vi "main_display.vi"() -> ()   [LabVIEW 2021]
uses:
  <vilib>/Instr/_visa.llb/VISA Configure Serial Port (Instr).vi
  <vilib>/Utility/file.llb/Write Delimited Spreadsheet (DBL).vi
panel:
  out "read buffer":string
  in  "Save Data":bool
  out "Sensor 8":dbl(slide) scale=0.0..10.0
  out "Sensor 7":dbl(slide) scale=0.0..10.0
  out "Sensor 6":dbl(slide) scale=0.0..10.0
  out "Sensor 5":dbl(slide) scale=0.0..10.0
  out "Sensor 4":dbl(slide) scale=0.0..10.0
  out "Sensor 3":dbl(slide) scale=0.0..10.0
  out "Sensor 2":dbl(slide) scale=0.0..10.0
  out "Sensor 1":dbl(slide) scale=0.0..10.0
  out "Output":dbl[](array[numeric])
  in  "file path (dialog if empty)":path
  out "Read time (ms)":u32
  in  "stop":bool
  in  "VISA resource name":refnum<visa-resource-name>
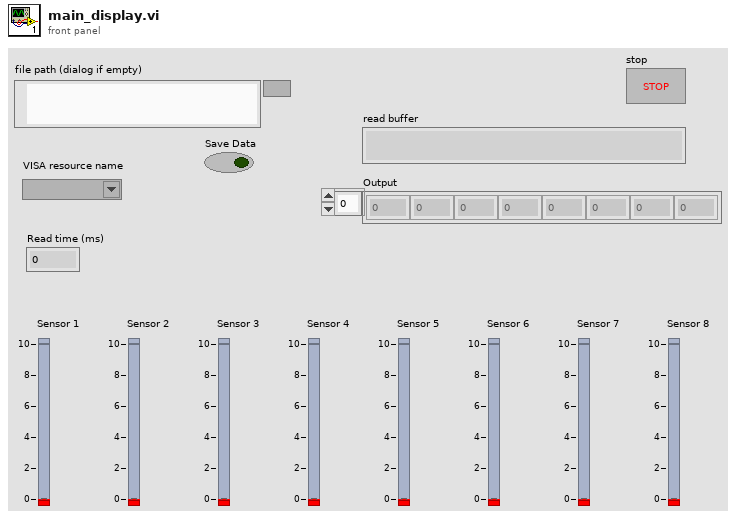
[diagram p1: front panel]
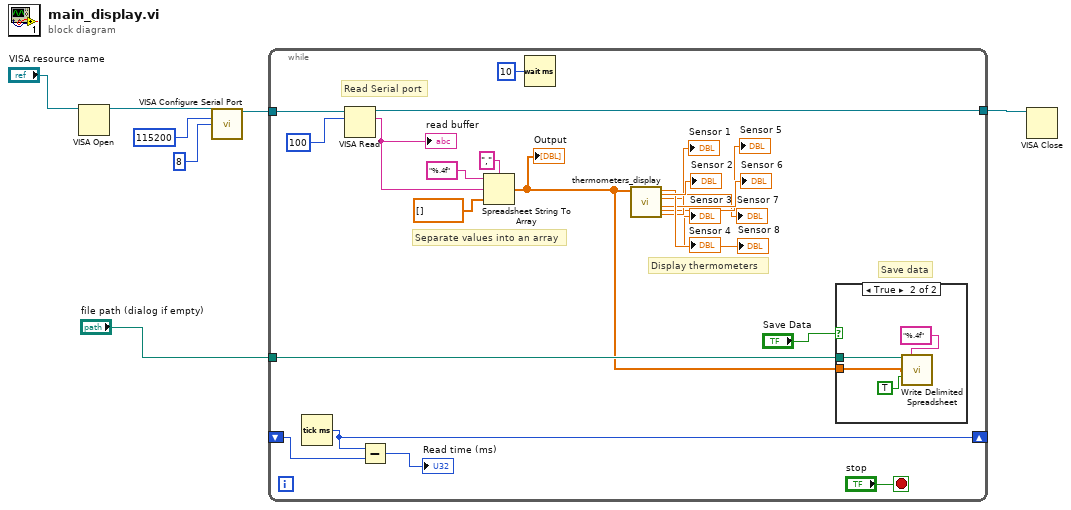
[diagram p0: block diagram]
diagram:
  n1 = VISA Open(VISA resource name="VISA resource name") -> (VISA resource name=w3:refnum<visa-resource-name>)  [unwired: 4 in, 1 out]
  n2 = call-poly "VISA Configure Serial Port"("VISA resource name"=w3, "baud rate (9600)"=u32 115200, "data bits (8)"=u16 8) -> ("VISA resource name out"=w5:refnum<visa-resource-name>)  [unwired: 11 in, 1 out]
  n3 = while {
    tunnel: w5 -> [w27]
    tunnel: [w28] -> w4
    shift-right: [w25] -> _
    shift-left: _ -> [w24]
    tunnel: "file path (dialog if empty)" -> [w22]
    stop <- "stop" stop-if-true
    # "Display thermometers"
    # "Save data"
    # "Separate values into an array"
    # "Read Serial port"
    n4 = Tick Count (ms)() -> (millisecond timer value=w25:u32)
    n5 = VISA Read(VISA resource name=w27, byte count=u32 100) -> (VISA resource name out=w28:refnum<visa-resource-name>, read buffer=w21:string)  [unwired: 1 in, 2 out]
    "read buffer" <- w21
    n6 = Subtract(x=w25, y=w24) -> (x-y=→"Read time (ms)":u32)
    n7 = Spreadsheet String To Array(delimiter (Tab)=",", format string="%.4f", spreadsheet string=w21, array type (2D Dbl)=dbl[] []) -> (array=w9:dbl[])
    "Output" <- w9
    n8 = Wait (ms)(milliseconds to wait=u32 10) -> ()  [unwired: 1 out]
    n9 = call "thermometers_display.vi"("array type (2D Dbl)"=w9) -> ("Sensor 1"=→"Sensor 1":dbl, "Sensor 6"=→"Sensor 6":dbl, "Sensor 4"=→"Sensor 4":dbl, "Sensor 8"=→"Sensor 8":dbl, "Sensor 5"=→"Sensor 5":dbl, "Sensor 2"=→"Sensor 2":dbl, "Sensor 3"=→"Sensor 3":dbl, "Sensor 7"=→"Sensor 7":dbl)  [unwired: 3 in]
    n10 = case shown="True" "Save Data" {
      tunnel: w22 -> [_ w32]
      tunnel: w9 -> [_ w31]
      frame False {
      }
      frame True {
        n11 = call-poly <vilib>:"Write Delimited Spreadsheet.vi"("file path (dialog if empty)"=w32, "format (%.3f)"="%.4f", "1D data"=w31, "append to file? (new file:F)"=TRUE) -> ()  [unwired: 10 in, 2 out]
      }
    }
  }
  n12 = VISA Close(VISA resource name=w4) -> ()  [unwired: 1 in, 1 out]
